vi "Initialize.vi"(8 "error in (no error)":errorcluster, 9 "Reset (f)":bool, 10 "IdQuery (f)":bool, 11 "IVI_Class in":refnum<class "IVI_Class.lvclass">) -> (0 "error out":errorcluster, 3 "IVI_Class out":refnum<class "IVI_Class.lvclass">)   [LabVIEW 2018, in "ScopePlugins.lvlib" / "IVI_Class.lvclass"]
uses:
  IVI_Class.lvclass
  Y:/Projects/PMUCal/Modules/Scope/ScopePlugins/ScopePluginBaseClass/ScopePluginsBase.lvclass
  ScopePluginBaseClass/ScopePluginsBase.lvclass/ScopePluginsBase.ctl
  ScopePluginBaseClass/Accessors/Read Handle.vi
  ScopePluginBaseClass/Accessors/Write Handle.vi
  ScopePluginBaseClass/Accessors/Write Connected.vi
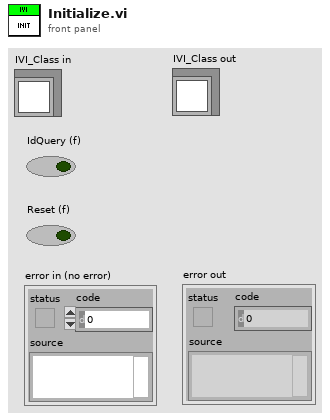
[diagram p1: front panel]
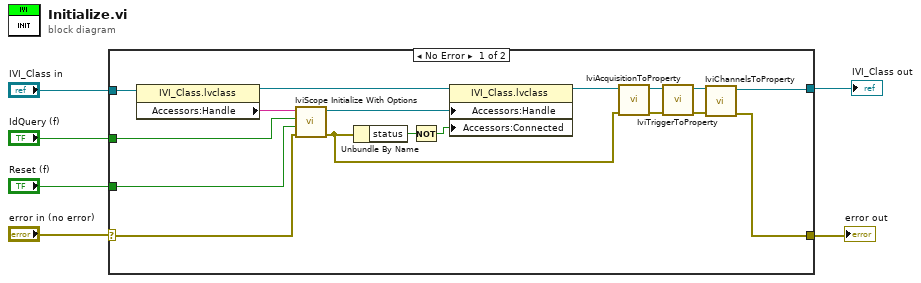
[diagram p0: block diagram]
diagram:
  n1 = case shown="No Error" "error in (no error)" {
    selector: "error in (no error)" -> [w19 w24]
    tunnel: "IVI_Class in" -> [w23 w25]
    tunnel: "IdQuery (f)" -> [w21 _]
    tunnel: "Reset (f)" -> [w20 _]
    tunnel: [w9 w25] -> w2
    tunnel: [w7 w24] -> w1
    frame No Error {
      n2 = property class="IVI_Class.lvclass"(reference=w23) -> (reference out=w18:refnum<class "IVI_Class.lvclass">, "Accessors:Handle"=w22:string)  [unwired: 1 in, 1 out]
      n3 = call <vilib>:"IviScope Initialize With Options.vi"("error in (no error)"=w19, "reset device (True)"=w20, "id query (True)"=w21, "logical name (\"SampleScope\")"=w22) -> ("error out"=w13:errorcluster, "instrument handle out"=w15:refnum<k15>)  [unwired: 6 in]
      n4 = Unbundle By Name(w13) -> ("status"=w17:bool)
      n5 = Not(x=w17) -> (.not. x?=w16:bool)
      n6 = property class="IVI_Class.lvclass"(reference=w18, "Accessors:Handle"=w15, "Accessors:Connected"=w16) -> (reference out=w14:refnum<class "IVI_Class.lvclass">)  [unwired: 1 in, 1 out]
      n7 = call "IviAcquisitionToProperty.vi"("error in (no error)"=w13, "IVI_Class.lvclass"=w14) -> ("error out"=w11:errorcluster, "IVI_Class.lvclass"=w12:refnum<class "IVI_Class.lvclass">)  [unwired: 8 in]
      n8 = call "IviTriggerToProperty.vi"("error in (no error)"=w11, "IVI_Class.lvclass"=w12) -> ("error out"=w8:errorcluster, "IVI_Class.lvclass"=w10:refnum<class "IVI_Class.lvclass">)  [unwired: 8 in]
      n9 = call "IviChannelsToProperty.vi"("error in (no error)"=w8, "IVI_Class.lvclass"=w10) -> ("error out"=w7:errorcluster, "IVI_Class.lvclass"=w9:refnum<class "IVI_Class.lvclass">)  [unwired: 8 in]
    }
    frame Error {
    }
  }
  "error out" <- w1
  "IVI_Class out" <- w2
